vi "GitGetFullHash.vi"(8 "error in (no error)":errorcluster, 9 "Directory":path=path "", 10 "Partial Hash":string, 11 "Git exec":string="git") -> (0 "error out":errorcluster, 1 "Directory out":path, 2 "Full Hash":string, 3 "Git exec out":string="git")   [LabVIEW 2013]
uses:
  GitCmd.vi
  <vilib>/dlg_ctls.llb/Space Constant.vi
  <vilib>/Utility/error.llb/General Error Handler.vi
  GitUtils/PathtoDirPath.vi
  <vilib>/Platform/system.llb/System Exec.vi
  <vilib>/Utility/error.llb/Error Cluster From Error Code.vi
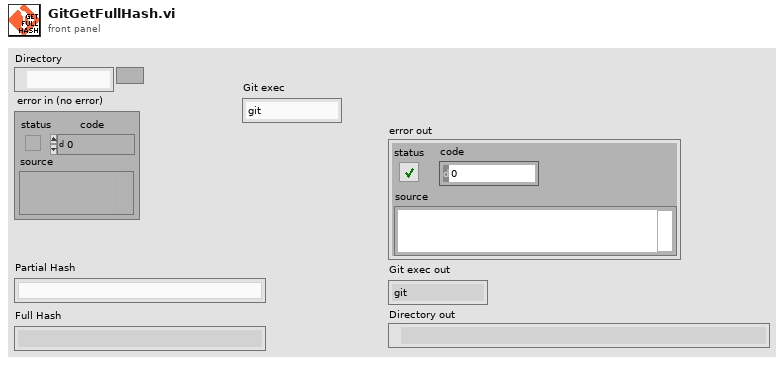
[diagram p1: front panel]
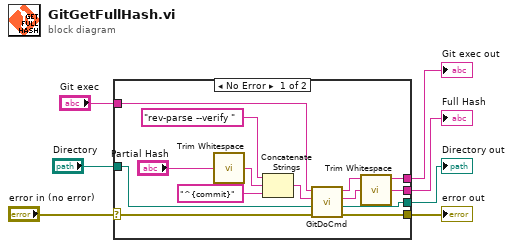
[diagram p0: block diagram]
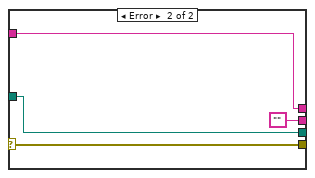
[diagram p2: hidden frame]
diagram:
  n1 = case shown="No Error" "error in (no error)" {
    selector: "error in (no error)" -> [w17 w23]
    tunnel: "Git exec" -> [w13 w21]
    tunnel: "Directory" -> [w16 w22]
    tunnel: [w15 ""] -> w5
    tunnel: [w20 w23] -> w4
    tunnel: [w19 w22] -> w2
    tunnel: [w18 w21] -> w1
    frame No Error {
      n2 = call <vilib>:"Trim Whitespace.vi"("string"="Partial Hash") -> ("trimmed string"=w12:string)  [unwired: 1 in]
      n3 = Concatenate Strings("rev-parse --verify " ("string"), w12, "^{commit}" ("string")) -> (w9:string)
      n4 = call "GitDoCmd.vi"("error in (no error)"=w17, "Working Path"=w16, "Git command"=w9, "Git exec"=w13) -> ("error out"=w20:errorcluster, "Working Path out"=w19:path, "Returned stdout"=w14:string, "Git exec out"=w18:string)  [unwired: 3 in]
      n5 = call <vilib>:"Trim Whitespace.vi"("string"=w14) -> ("trimmed string"=w15:string)  [unwired: 1 in]
    }
    frame Error {
    }
  }
  "Full Hash" <- w5
  "error out" <- w4
  "Git exec out" <- w1
  "Directory out" <- w2
